vi "Read-CompCoeffs.vi"(7 "Slave Address (7-bit)":u8, 8 "error in (no error)":errorcluster, 11 "I2C Ref Out in":T1) -> (0 "error out":errorcluster, 2 "Comp Coeffs Out":T9 {"dig_H6" format="%0d"; "dig_H5" format="%0d"; "dig_H4" format="%0d"; "dig_H3" format="%0d"; "dig_H2" format="%0d"; "dig_H1" format="%0d"; "dig_P9" format="%0d"; "dig_P8" format="%0d"; "dig_P7" format="%0d"; "dig_P6" format="%0d"; "dig_P5" format="%0d"; "dig_P4" format="%0d"; "dig_P3" format="%0d"; "dig_P2" format="%0d"; "dig_P1" format="%0d"; "dig_T3" format="%0d"; "dig_T2" format="%0d"; "dig_T1" format="%0d"}, 3 "I2C Ref Out out":T1)   [LabVIEW 2015]
uses:
  calib_data.ctl
  <vilib>/myRIO/Instrument Drivers/Onboard IO/I2C/typedefs/I2C Reference.ctl
  <vilib>/myRIO/Common/Instrument Driver Framework/Utilities/typedefs/myRIO Generic Hardware Reference.ctl
  <vilib>/myRIO/Common/Instrument Driver Framework/Utilities/typedefs/Hardware Version Enum.ctl
  <vilib>/myRIO/Common/Instrument Driver Framework/Utilities/typedefs/myRIO v1.0 Reference.ctl
  <vilib>/myRIO/Common/Instrument Driver Framework/Utilities/typedefs/Generic FPGA Reference.ctl
  <vilib>/myRIO/Common/Instrument Driver Framework/myRIO v1.0/I2C/typedefs/I2C Channels Enum.ctl
  <vilib>/myRIO/Instrument Drivers/Onboard IO/I2C/typedefs/I2C Configuration.ctl
  <vilib>/myRIO/Instrument Drivers/Onboard IO/I2C/typedefs/I2C Transfer Rate.ctl
  <vilib>/Utility/error.llb/Error Cluster From Error Code.vi
  <vilib>/myRIO/Common/Instrument Driver Framework/myRIO v1.0/I2C/vis/myRIO v1.0 Write I2C.vi
  <vilib>/myRIO/Common/Instrument Driver Framework/myRIO v1.0/I2C/vis/myRIO v1.0 Read I2C.vi
  <vilib>/myRIO/Instrument Drivers/Onboard IO/I2C/I2C.lvlib
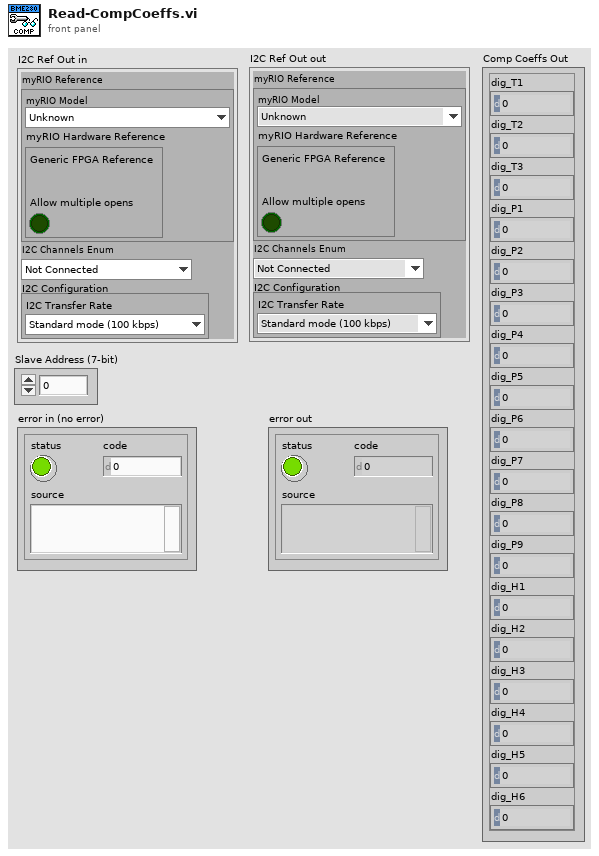
[diagram p1: front panel]
types:
  T1 = typedef "I2C.lvlib/I2C Reference.ctl" = cluster{"myRIO Reference":T2, "I2C Channels Enum":T6, "I2C Configuration":T7}
  T2 = typedef "myRIO Generic Hardware Reference.ctl" = cluster{"myRIO Model":T3, "myRIO Hardware Reference":T4}
  T3 = typedef "Hardware Version Enum.ctl" = enum16{"Unknown", "myRIO-1900", "myRIO-1950", "roboRIO"}
  T4 = typedef "myRIO v1.0 Reference.ctl" = cluster{"Generic FPGA Reference":T5, "Allow multiple opens":bool}
  T5 = typedef "Generic FPGA Reference.ctl" = refnum<k20>
  T6 = typedef "I2C Channels Enum.ctl" = enum16{"Not Connected", "A/I2C", "B/I2C", "I2C/I2C"}
  T7 = typedef "I2C.lvlib/I2C Configuration.ctl" = cluster{"I2C Transfer Rate":T8}
  T8 = typedef "I2C.lvlib/I2C Transfer Rate.ctl" = enum16{"Standard mode (100 kbps)", "Fast mode (400 kbps)"}
  T9 = typedef "calib_data.ctl" = cluster{"dig_T1":u16, "dig_T2":i16, "dig_T3":i16, "dig_P1":u16, "dig_P2":i16, "dig_P3":i16, "dig_P4":i16, "dig_P5":i16, "dig_P6":i16, "dig_P7":i16, "dig_P8":i16, "dig_P9":i16, "dig_H1":u8, "dig_H2":i16, "dig_H3":u8, "dig_H4":i16, "dig_H5":i16, "dig_H6":i8}
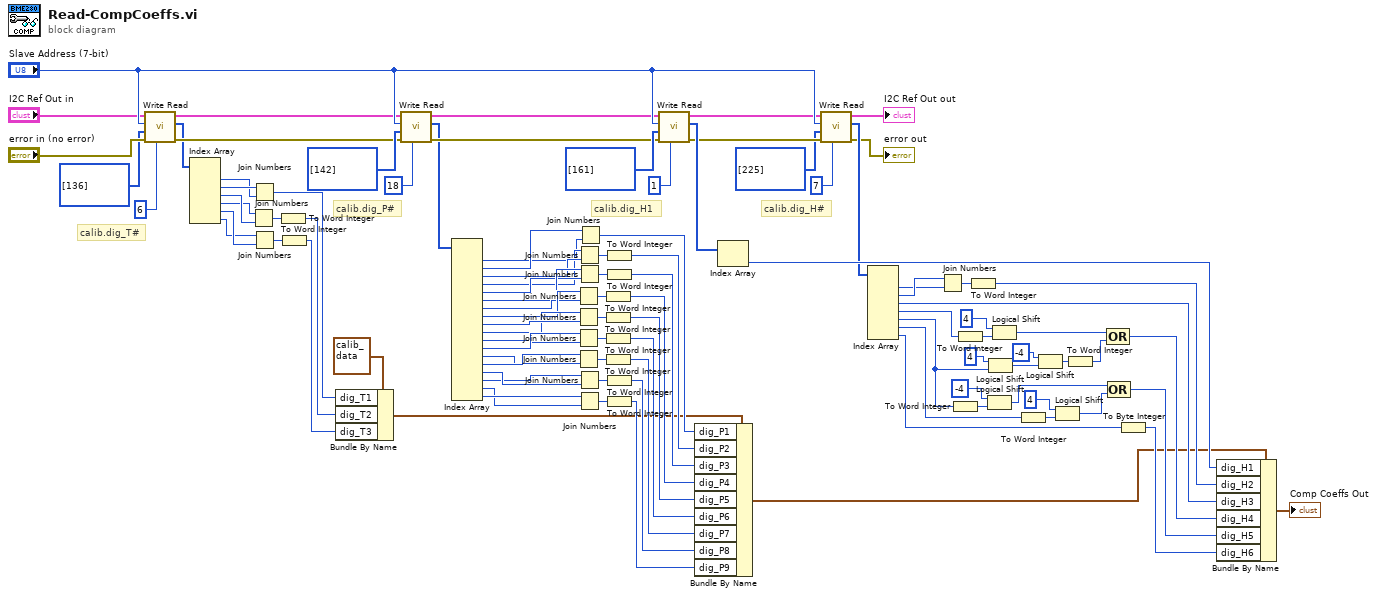
[diagram p0: block diagram]
diagram:
  # "calib.dig_H#"
  # "calib.dig_H1"
  # "calib.dig_P#"
  # "calib.dig_T#"
  n1 = call <vilib>:"Write Read.vi"("Byte Count"=u32 6, "error in (no error)"="error in (no error)", "Bytes to Write"=u8[] [136], "Slave Address (7-bit)"="Slave Address (7-bit)", "I2C Ref In"="I2C Ref Out in") -> ("error out"=w15:errorcluster, "Bytes Read"=w5:u8[], "I2C Ref Out"=w14:T1)  [unwired: 3 in]
  n2 = Index Array(array=w5) -> (element #1=w6:u8, element #2=w7:u8, element #3=w10:u8, element #4=w9:u8, element #5=w13:u8, element #6=w12:u8)  [unwired: 6 in]
  n3 = Join Numbers(hi=w9, lo=w10) -> ((hi.lo)=w8:u16)
  n4 = Join Numbers(hi=w7, lo=w6) -> ((hi.lo)=w80:u16)
  n5 = Join Numbers(hi=w12, lo=w13) -> ((hi.lo)=w11:u16)
  n6 = To Word Integer(number=w8) -> (16bit integer=w81:i16)
  n7 = To Word Integer(number=w11) -> (16bit integer=w82:i16)
  n8 = Bundle By Name(cluster=T9 {"dig_T1"=0, "dig_T2"=0, "dig_T3"=0, "dig_P1"=0, "dig_P2"=0, "dig_P3"=0, "dig_P4"=0, "dig_P5"=0, "dig_P6"=0, "dig_P7"=0, "dig_P8"=0, "dig_P9"=0, "dig_H1"=0, "dig_H2"=0, "dig_H3"=0, "dig_H4"=0, "dig_H5"=0, "dig_H6"=0}, "dig_T1"=w80, "dig_T2"=w81, "dig_T3"=w82) -> (w83:T9)
  n9 = call <vilib>:"Write Read.vi"("Byte Count"=u32 18, "error in (no error)"=w15, "Bytes to Write"=u8[] [142], "Slave Address (7-bit)"="Slave Address (7-bit)", "I2C Ref In"=w14) -> ("error out"=w46:errorcluster, "Bytes Read"=w18:u8[], "I2C Ref Out"=w45:T1)  [unwired: 3 in]
  n10 = Index Array(array=w18) -> (element #1=w19:u8, element #2=w20:u8, element #3=w23:u8, element #4=w22:u8, element #5=w31:u8, element #6=w32:u8, element #7=w33:u8, element #8=w34:u8, element #9=w36:u8, element #10=w35:u8, element #11=w37:u8, element #12=w38:u8, element #13=w39:u8, element #14=w40:u8, element #15=w42:u8, element #16=w41:u8, element #17=w43:u8, element #18=w44:u8)  [unwired: 18 in]
  n11 = Join Numbers(hi=w34, lo=w33) -> ((hi.lo)=w25:u16)
  n12 = Join Numbers(hi=w35, lo=w36) -> ((hi.lo)=w26:u16)
  n13 = Join Numbers(hi=w38, lo=w37) -> ((hi.lo)=w27:u16)
  n14 = Join Numbers(hi=w40, lo=w39) -> ((hi.lo)=w28:u16)
  n15 = Join Numbers(hi=w22, lo=w23) -> ((hi.lo)=w21:u16)
  n16 = Join Numbers(hi=w32, lo=w31) -> ((hi.lo)=w24:u16)
  n17 = Join Numbers(hi=w41, lo=w42) -> ((hi.lo)=w29:u16)
  n18 = Join Numbers(hi=w44, lo=w43) -> ((hi.lo)=w30:u16)
  n19 = Join Numbers(hi=w20, lo=w19) -> ((hi.lo)=w84:u16)
  n20 = To Word Integer(number=w25) -> (16bit integer=w87:i16)
  n21 = To Word Integer(number=w26) -> (16bit integer=w88:i16)
  n22 = To Word Integer(number=w27) -> (16bit integer=w89:i16)
  n23 = To Word Integer(number=w28) -> (16bit integer=w90:i16)
  n24 = To Word Integer(number=w21) -> (16bit integer=w86:i16)
  n25 = To Word Integer(number=w24) -> (16bit integer=w85:i16)
  n26 = To Word Integer(number=w29) -> (16bit integer=w91:i16)
  n27 = To Word Integer(number=w30) -> (16bit integer=w92:i16)
  n28 = call <vilib>:"Write Read.vi"("Byte Count"=u32 1, "error in (no error)"=w46, "Bytes to Write"=u8[] [161], "Slave Address (7-bit)"="Slave Address (7-bit)", "I2C Ref In"=w45) -> ("error out"=w52:errorcluster, "Bytes Read"=w55:u8[], "I2C Ref Out"=w51:T1)  [unwired: 3 in]
  n29 = Bundle By Name(cluster=w83, "dig_P1"=w84, "dig_P2"=w86, "dig_P3"=w85, "dig_P4"=w87, "dig_P5"=w88, "dig_P6"=w89, "dig_P7"=w90, "dig_P8"=w91, "dig_P9"=w92) -> (w93:T9)
  n30 = Index Array(array=w55) -> (element=w94:u8)  [unwired: 1 in]
  n31 = call <vilib>:"Write Read.vi"("Byte Count"=u32 7, "error in (no error)"=w52, "Bytes to Write"=u8[] [225], "Slave Address (7-bit)"="Slave Address (7-bit)", "I2C Ref In"=w51) -> ("error out"=→"error out":errorcluster, "Bytes Read"=w56:u8[], "I2C Ref Out"=→"I2C Ref Out out":T1)  [unwired: 3 in]
  n32 = Index Array(array=w56) -> (element #1=w57:u8, element #2=w58:u8, element #3=w96:u8, element #4=w61:u8, element #5=w73:u8, element #6=w71:u8, element #7=w70:u8)  [unwired: 7 in]
  n33 = Join Numbers(hi=w58, lo=w57) -> ((hi.lo)=w59:u16)
  n34 = To Word Integer(number=w73) -> (16bit integer=w66:i16)
  n35 = To Word Integer(number=w61) -> (16bit integer=w62:i16)
  n36 = To Word Integer(number=w59) -> (16bit integer=w95:i16)
  n37 = Logical Shift(y=i16 -4, x=w66) -> (x << y=w72:i16)
  n38 = Logical Shift(y=i16 4, x=w73) -> (x << y=w75:u8)
  n39 = Logical Shift(y=i16 4, x=w62) -> (x << y=w69:i16)
  n40 = To Word Integer(number=w71) -> (16bit integer=w65:i16)
  n41 = Logical Shift(y=i16 -4, x=w75) -> (x << y=w77:u8)
  n42 = Logical Shift(y=i16 4, x=w65) -> (x << y=w68:i16)
  n43 = To Word Integer(number=w77) -> (16bit integer=w78:i16)
  n44 = Compound Arithmetic op=OR(w69, w78) -> (w97:i16)
  n45 = Compound Arithmetic op=OR(w72, w68) -> (w98:i16)
  n46 = To Byte Integer(number=w70) -> (8bit integer=w99:i8)
  n47 = Bundle By Name(cluster=w93, "dig_H1"=w94, "dig_H2"=w95, "dig_H3"=w96, "dig_H4"=w97, "dig_H5"=w98, "dig_H6"=w99) -> (→"Comp Coeffs Out":T9)
